vi "Set Measurement.vi"(6 "Escala":dbl, 8 "error in (no error)":errorcluster, 9 "Range ON/OFF":bool, 10 "Grandeza Elétrica":string, 11 "189 in":refnum<class "189.lvclass">) -> (0 "error out":errorcluster, 3 "189 out":refnum<class "189.lvclass">)   [LabVIEW 2015, in "189.lvclass"]
uses:
  189.lvclass
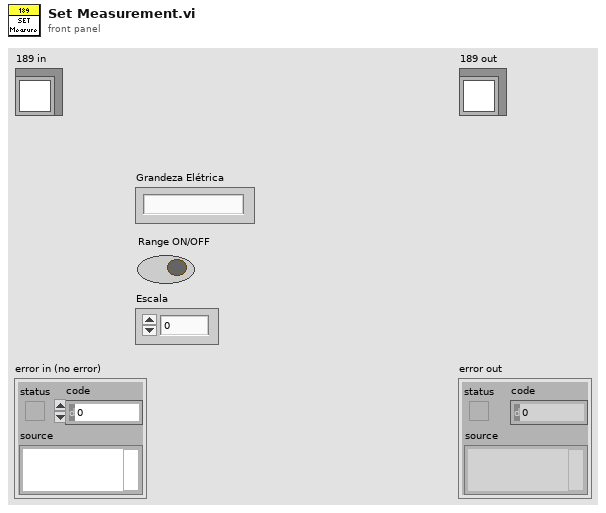
[diagram p1: front panel]
types:
  T1 = enum16{"5 V", "50 V", "500 V", "1000 V", "50 mV", "500 mV", "5000 mV", "500 Ohms", "5 kOhms", "50 kOhms", "500 kOhms", "5 MOhms", "30 MOhms", "500 MOhms", "1 uF", "10 uF", "100 uF", "1 mF", "10 mF", "50 mF", "5 A", "10 A", "50 mA", "500 mA", "500 uA", "5000 uA"}[]
  T2 = enum16{"5 V", "50 V", "500 V", "1000 V", "50 mV", "500 mV", "5000 mV", "500 Ohms", "5 kOhms", "50 kOhms", "500 kOhms", "5 MOhms", "30 MOhms", "500 MOhms", "1 uF", "10 uF", "100 uF", "1 mF", "10 mF", "50 mF", "5 A", "10 A", "50 mA", "500 mA", "500 uA", "5000 uA"}
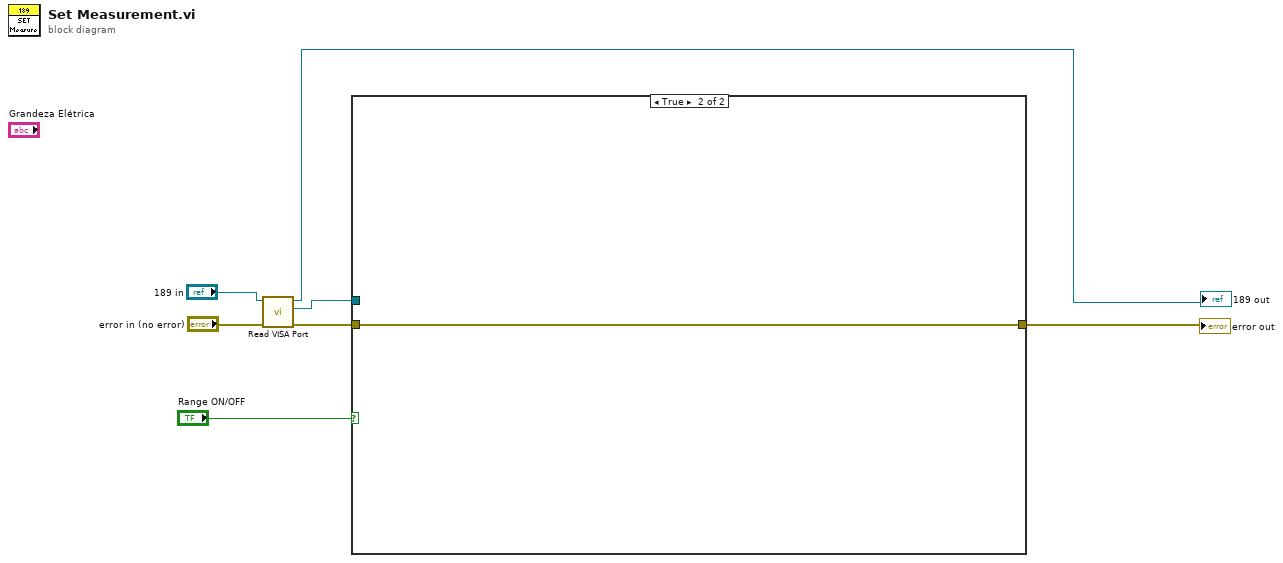
[diagram p0: block diagram]
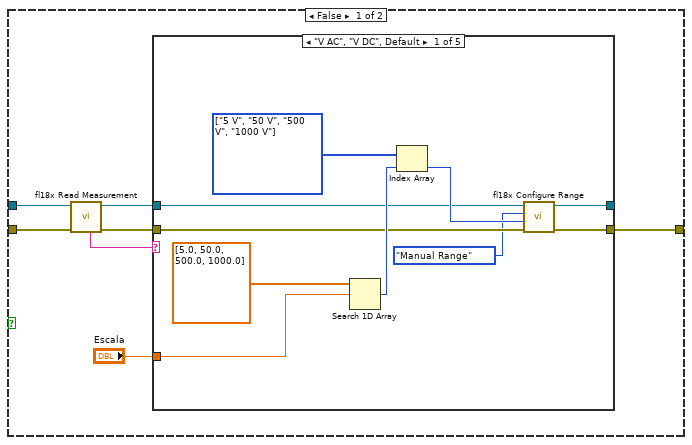
[diagram p2: hidden frame]
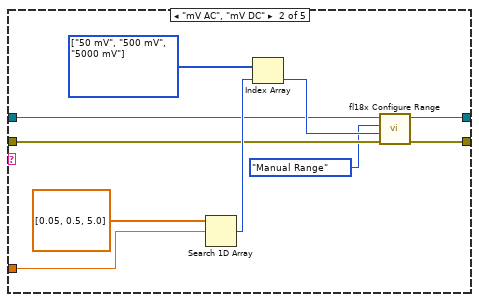
[diagram p3: hidden frame]
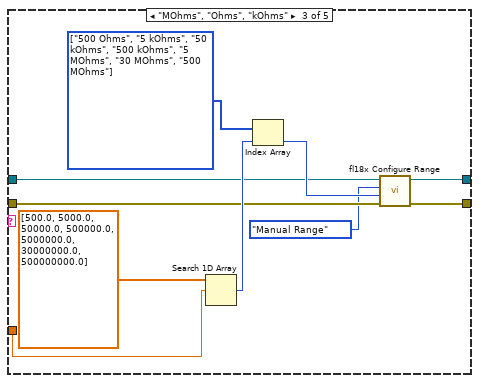
[diagram p4: hidden frame]
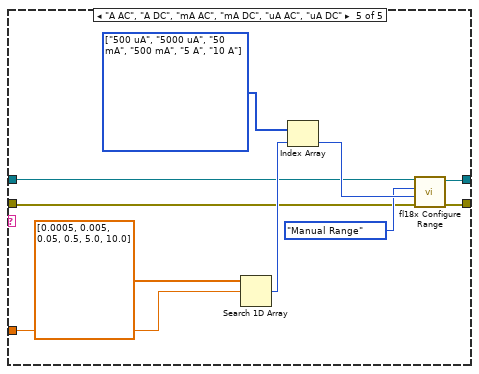
[diagram p6: hidden frame]
diagram:
  n1 = call-dynamic "Read VISA Port.vi"("error in (no error)"="error in (no error)", "Device in"="189 in") -> ("error out"=w4:errorcluster, "VISA Port"=w5:refnum<visa-resource-name>, "Device out"=→"189 out":refnum<class "189.lvclass">)  [unwired: 7 in]
  n2 = case shown="True" "Range ON/OFF" {
    tunnel: w5 -> [w14 _]
    tunnel: w4 -> [w13 w57]
    tunnel: [w8 w57] -> w3
    frame False {
      n3 = call <instrlib>:"fl18x Read Measurement.vi"("error in (no error)"=w13, "VISA session"=w14) -> ("error out"=w10:errorcluster, "dup VISA session"=w11:refnum<visa-resource-name>, "Unidade"=w12:string)  [unwired: 5 in, 2 out]
      n4 = case shown="\"V AC\", \"V DC\", Default" w12 {
        tunnel: w11 -> [w21 w31 w41 w46 w52]
        tunnel: w10 -> [w20 w30 w40 w45 w51]
        tunnel: [w18 w28 w38 w46 w50] -> _
        tunnel: [w17 w27 w37 w45 w49] -> w8
        tunnel: "Escala" -> [w15 w25 w35 _ w47]
        frame "V AC", "V DC", Default {
          w24 = T1 [enum."5 V", enum."50 V", enum."500 V", enum."1000 V"] items=["5 V", "50 V", "500 V", "1000 V", "50 mV", "500 mV", "5000 mV", "500 Ohms", "5 kOhms", "50 kOhms", "500 kOhms", "5 MOhms", "30 MOhms", "500 MOhms", "1 uF", "10 uF", "100 uF", "1 mF", "10 mF", "50 mF", "5 A", "10 A", "50 mA", "500 mA", "500 uA", "5000 uA"]
          n5 = Search 1D Array(1D array=dbl[] [5.0, 50.0, 500.0, 1000.0], element=w15) -> (index of element=w23:i32)  [unwired: 1 in]
          n6 = Index Array(array=w24, index=w23) -> (element=w22:T2)
          n7 = call <instrlib>:"fl18x Configure Range.vi"("error in (no error)"=w20, "Range (5V)"=w22, "Function (Exit Manual)"=enum16{"Exit Manual", "Manual Range"}."Manual Range", "VISA session"=w21) -> ("error out"=w17:errorcluster, "dup VISA session"=w18:refnum<visa-resource-name>)  [unwired: 6 in]
        }
        frame "mV AC", "mV DC" {
          w34 = T1 [enum."50 mV", enum."500 mV", enum."5000 mV"] items=["5 V", "50 V", "500 V", "1000 V", "50 mV", "500 mV", "5000 mV", "500 Ohms", "5 kOhms", "50 kOhms", "500 kOhms", "5 MOhms", "30 MOhms", "500 MOhms", "1 uF", "10 uF", "100 uF", "1 mF", "10 mF", "50 mF", "5 A", "10 A", "50 mA", "500 mA", "500 uA", "5000 uA"]
          n8 = Search 1D Array(1D array=dbl[] [0.05, 0.5, 5.0], element=w25) -> (index of element=w33:i32)  [unwired: 1 in]
          n9 = Index Array(array=w34, index=w33) -> (element=w32:T2)
          n10 = call <instrlib>:"fl18x Configure Range.vi"("error in (no error)"=w30, "Range (5V)"=w32, "Function (Exit Manual)"=enum16{"Exit Manual", "Manual Range"}."Manual Range", "VISA session"=w31) -> ("error out"=w27:errorcluster, "dup VISA session"=w28:refnum<visa-resource-name>)  [unwired: 6 in]
        }
        frame "MOhms", "Ohms", "kOhms" {
          w44 = T1 [enum."500 Ohms", enum."5 kOhms", enum."50 kOhms", enum."500 kOhms", enum."5 MOhms", enum."30 MOhms", enum."500 MOhms"] items=["5 V", "50 V", "500 V", "1000 V", "50 mV", "500 mV", "5000 mV", "500 Ohms", "5 kOhms", "50 kOhms", "500 kOhms", "5 MOhms", "30 MOhms", "500 MOhms", "1 uF", "10 uF", "100 uF", "1 mF", "10 mF", "50 mF", "5 A", "10 A", "50 mA", "500 mA", "500 uA", "5000 uA"]
          n11 = Search 1D Array(1D array=dbl[] [500.0, 5000.0, 50000.0, 500000.0, 5000000.0, 30000000.0, 500000000.0], element=w35) -> (index of element=w43:i32)  [unwired: 1 in]
          n12 = Index Array(array=w44, index=w43) -> (element=w42:T2)
          n13 = call <instrlib>:"fl18x Configure Range.vi"("error in (no error)"=w40, "Range (5V)"=w42, "Function (Exit Manual)"=enum16{"Exit Manual", "Manual Range"}."Manual Range", "VISA session"=w41) -> ("error out"=w37:errorcluster, "dup VISA session"=w38:refnum<visa-resource-name>)  [unwired: 6 in]
        }
        frame "Hz" {
        }
        frame "A AC", "A DC", "mA AC", "mA DC", "uA AC", "uA DC" {
          w56 = T1 [enum."500 uA", enum."5000 uA", enum."50 mA", enum."500 mA", enum."5 A", enum."10 A"] items=["5 V", "50 V", "500 V", "1000 V", "50 mV", "500 mV", "5000 mV", "500 Ohms", "5 kOhms", "50 kOhms", "500 kOhms", "5 MOhms", "30 MOhms", "500 MOhms", "1 uF", "10 uF", "100 uF", "1 mF", "10 mF", "50 mF", "5 A", "10 A", "50 mA", "500 mA", "500 uA", "5000 uA"]
          n14 = Search 1D Array(1D array=dbl[] [0.0005, 0.005, 0.05, 0.5, 5.0, 10.0], element=w47) -> (index of element=w55:i32)  [unwired: 1 in]
          n15 = Index Array(array=w56, index=w55) -> (element=w54:T2)
          n16 = call <instrlib>:"fl18x Configure Range.vi"("error in (no error)"=w51, "Range (5V)"=w54, "Function (Exit Manual)"=enum16{"Exit Manual", "Manual Range"}."Manual Range", "VISA session"=w52) -> ("error out"=w49:errorcluster, "dup VISA session"=w50:refnum<visa-resource-name>)  [unwired: 6 in]
        }
      }
    }
    frame True {
    }
  }
  "error out" <- w3
